vi "Coerce to shortest distance.vi"(9 "Angle 2":dbl, 10 "Angle 1":dbl) -> (2 "Shortest distance":dbl)   [LabVIEW 2020]
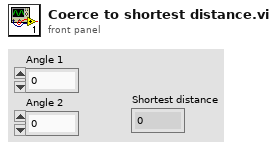
[diagram p1: front panel]
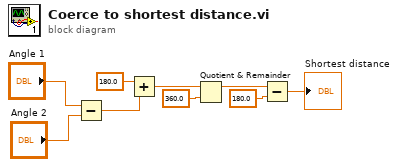
[diagram p0: block diagram]
diagram:
  n1 = Subtract(x="Angle 1", y="Angle 2") -> (x-y=w3:dbl)
  n2 = Add(x=180.0, y=w3) -> (x+y=w8:dbl)
  n3 = Quotient & Remainder(x=w8, y=360.0) -> (x-y*floor(x/y)=w5:dbl)  [unwired: 1 out]
  n4 = Subtract(x=w5, y=180.0) -> (x-y=→"Shortest distance":dbl)
